vi "SPL meter average testing.vi"() -> ()   [LabVIEW 2018]
uses:
  <vilib>/sound2/lvsound2.llb/Sound Input Read (DBL).vi
panel:
  in  "file path (use dialog)":path
  in  "stop":bool
  out "Waveform Chart":cluster{dbl}(graph)
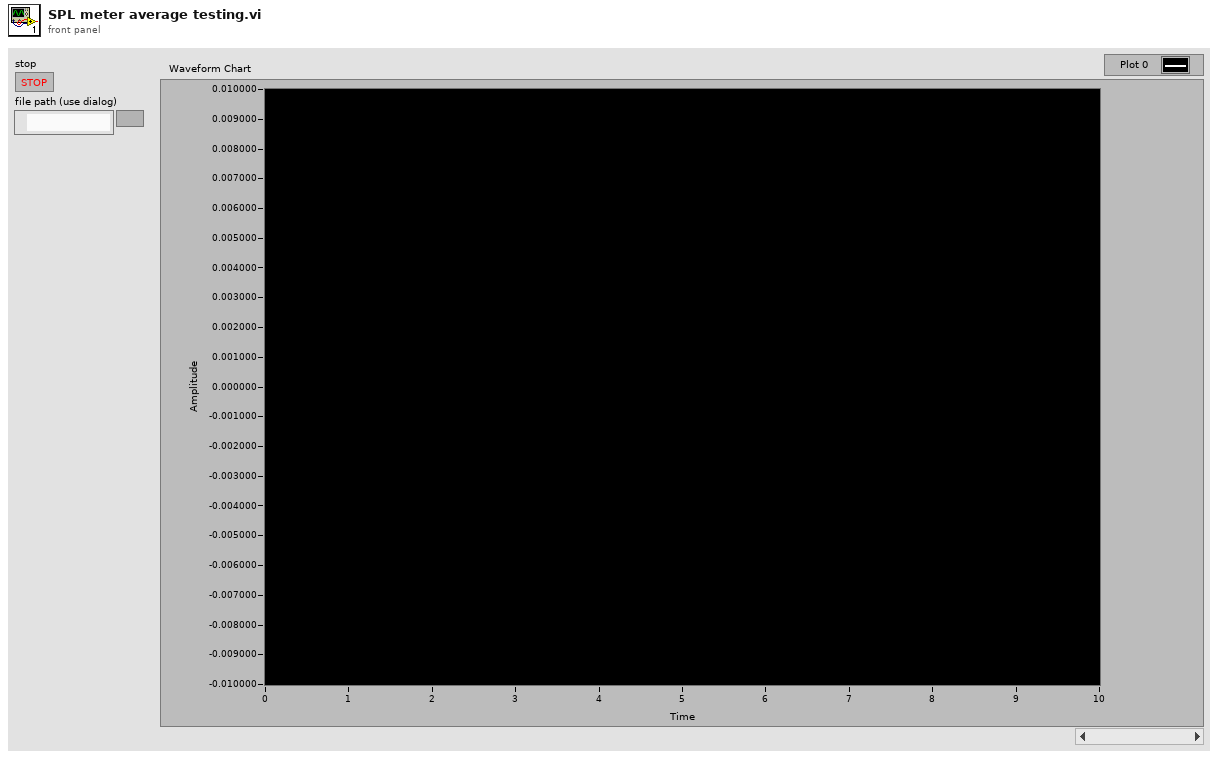
[diagram p1: front panel]
types:
  T1 = enum16{"open", "replace", "create", "open or create", "replace or create", "replace or create with confirmation"}
  T2 = typedef "Sound Input Task ID.ctl" = u32
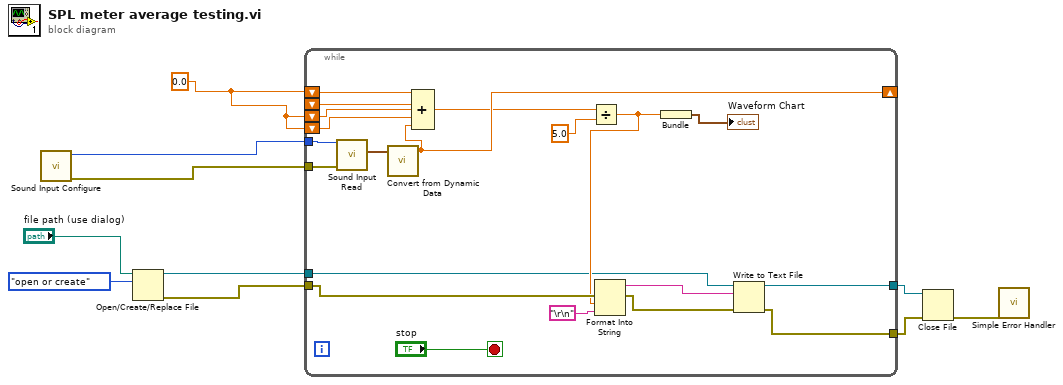
[diagram p0: block diagram]
diagram:
  w8 = 0.0
  n1 = call <vilib>:"Sound Input Configure.vi"() -> ("error out"=w10:errorcluster, "task ID"=w9:T2)  [unwired: 10 in]
  n2 = Open/Create/Replace File(file path (use dialog)="file path (use dialog)", operation (0:open)=T1."open or create") -> (refnum out=w1:refnum<file>, error out=w5:errorcluster)  [unwired: 4 in, 1 out]
  n3 = while {
    tunnel: w10 -> [w30]
    tunnel: w9 -> [w29]
    shift-right: [w24] -> _
    shift-left: w8 -> [w28]
    shift-left: w8 -> [w27]
    shift-left: w8 -> [w26]
    shift-left: w8 -> [w25]
    tunnel: w5 -> [w22]
    tunnel: [w19] -> w4
    tunnel: [w18] -> w3
    tunnel: w1 -> [w13]
    stop <- "stop" stop-if-true
    n4 = call-poly <vilib>:"Sound Input Read.vi"("error in (no error)"=w30, "task ID"=w29) -> ("data"=w11:waveform(dbl)[])  [unwired: 7 in, 2 out]
    n5 = call "Convert from Dynamic Data"("Dynamic Data Type"=w11) -> ("Scalar"=w24:dbl)  [unwired: 3 in]
    n6 = Compound Arithmetic op=ADD(w28, w27, w26, w25, w24) -> (w17:dbl)
    n7 = Divide(x=w17, y=5.0) -> (x/y=w14:dbl)
    n8 = Format Into String(error in=w22, w14, "\r\n") -> (resulting string=w20:string, error out=w21:errorcluster)  [unwired: 2 in]
    n9 = Bundle(w14) -> (→"Waveform Chart":cluster{dbl})  [unwired: 1 in]
    n10 = Write to Text File(file (use dialog)=w13, text=w20, error in=w21) -> (refnum out=w18:refnum<file>, error out=w19:errorcluster)  [unwired: 1 in, 1 out]
  }
  n11 = Close File(refnum=w3, error in=w4) -> (error out=w6:errorcluster)  [unwired: 1 out]
  n12 = call <vilib>:"Simple Error Handler.vi"("error in (no error)"=w6) -> ()  [unwired: 4 in, 5 out]
